vi "Default Path.vi"() -> (0 "Default Path data 2":path, 1 "Default Path data":path)   [LabVIEW 2011]
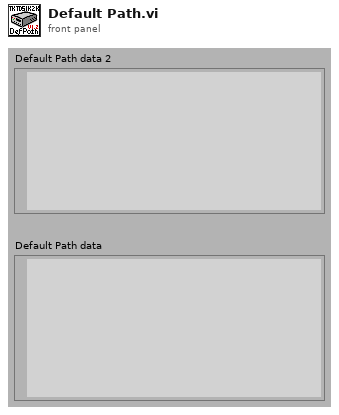
[diagram p1: front panel]
types:
  T1 = enum32{"invalid app kind", "Development System", "Run Time System", "Student Edition", "Embedded LabVIEW", "Evaluation", "Custom"}
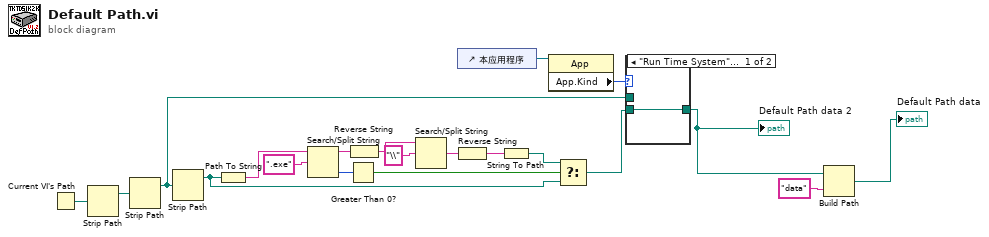
[diagram p0: block diagram]
diagram:
  n1 = Current VI's Path() -> (path=w20:path)
  n2 = Strip Path(path=w20) -> (stripped path=w16:path)  [unwired: 1 out]
  n3 = Strip Path(path=w16) -> (stripped path=w8:path)  [unwired: 1 out]
  n4 = Strip Path(path=w8) -> (stripped path=w3:path)  [unwired: 1 out]
  n5 = Path To String(path=w3) -> (string=w9:string)
  n6 = Search/Split String(string=w9, search string/char (-)=".exe" ("搜索字符串/字符(-)")) -> (substring before match=w14:string, offset of match=w7:i32)  [unwired: 1 in, 1 out]
  n7 = Greater Than 0?(x=w7) -> (x > 0?=w6:bool)
  n8 = Reverse String(1:w14) -> (0:w12:string)
  n9 = Search/Split String(string=w12, search string/char (-)="\\" ("搜索字符串/字符(-)")) -> (match + rest of string=w10:string)  [unwired: 1 in, 2 out]
  n10 = Reverse String(1:w10) -> (0:w11:string)
  n11 = control-ref of="本应用程序"() -> (w19:refnum<vi>)
  n12 = String To Path(string=w11) -> (path=w5:path)
  n13 = property class="App"(reference=w19) -> ("App.Kind"=w18:T1)  [unwired: 1 in, 2 out]
  n14 = Select(t=w5, s=w6, f=w3) -> (s? t:f=w4:path)
  n15 = case shown="\"Run Time System\", 默认" w18 {
    tunnel: w8 -> [_ w22]
    tunnel: [w21 w22] -> w1
    tunnel: w4 -> [w21 _]
    frame "Run Time System", Default {
    }
    frame "Development System" {
    }
  }
  "Default Path data 2" <- w1
  n16 = Build Path(base path=w1, name or relative path="data") -> (appended path=→"Default Path data":path)
